vi "匹配精确整型数示例.vi"() -> ()   [LabVIEW 2011]
uses:
  <vilib>/regexp/Match Regular Expression.xnode
panel:
  in  "整型数":i32
  out "匹配后偏移量":i32=8
  out "匹配之后":string="V，电流=11A。"
  out "所有匹配":string="212"
  out "匹配之前":string="电压="
  in  "字符串":string="电压=212V，电流=11A。"
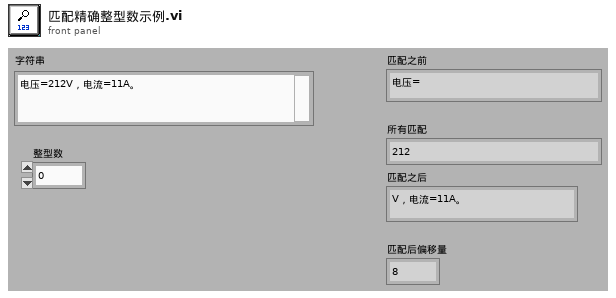
[diagram p1: front panel]
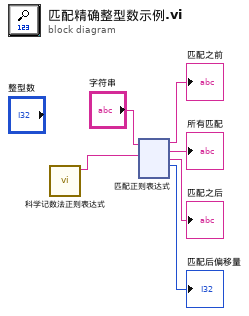
[diagram p0: block diagram]
diagram:
  n1 = call "科学记数法正则表达式.vi"() -> ("正则表达式"=w1:string)  [unwired: 10 in, 1 out]
  n2 = xnode "匹配正则表达式"("输入字符串"="字符串", "正则表达式"=w1) -> ("匹配之前"=→"匹配之前":string, "所有匹配"=→"所有匹配":string, "匹配之后"=→"匹配之后":string, "匹配后偏移量"=→"匹配后偏移量":i32)  [unwired: 4 in, 1 out]
